vi "SelfCal.vi"(8 "error in (no error)":errorcluster, 10 "gRPCid":T4, 11 "ctet_smu":T1) -> (0 "error out":errorcluster, 3 "ctet_smu out":T1)   [LabVIEW 2019, in "ctet_smu User Library.lvlib"]
uses:
  ctet_smu User Library.lvlib
  Servers/ctet_smu/gRPC lvSupport/Server API/typeDefs/grpcId.ctl
  Types/ctet_smu.ctl
  Servers/ctet_smu/ctet_smu Class/RPC Messages/measurementservice_SMUConfigResponse/measurementservice_SMUConfigResponse_Data.ctl
  Servers/ctet_smu/ctet_smu Class/RPC Messages/measurementservice_ErrorOut/measurementservice_ErrorOut_Data.ctl
  Servers/ctet_smu/ctet_smu Class/RPC Messages/measurementservice_SMUSelfCalResponse/measurementservice_SMUSelfCalResponse_Data.ctl
  Servers/ctet_smu/ctet_smu Class/ctet_smu.lvclass
  Servers/ctet_smu/gRPC lvSupport/gprc-lvsupport.lvlib
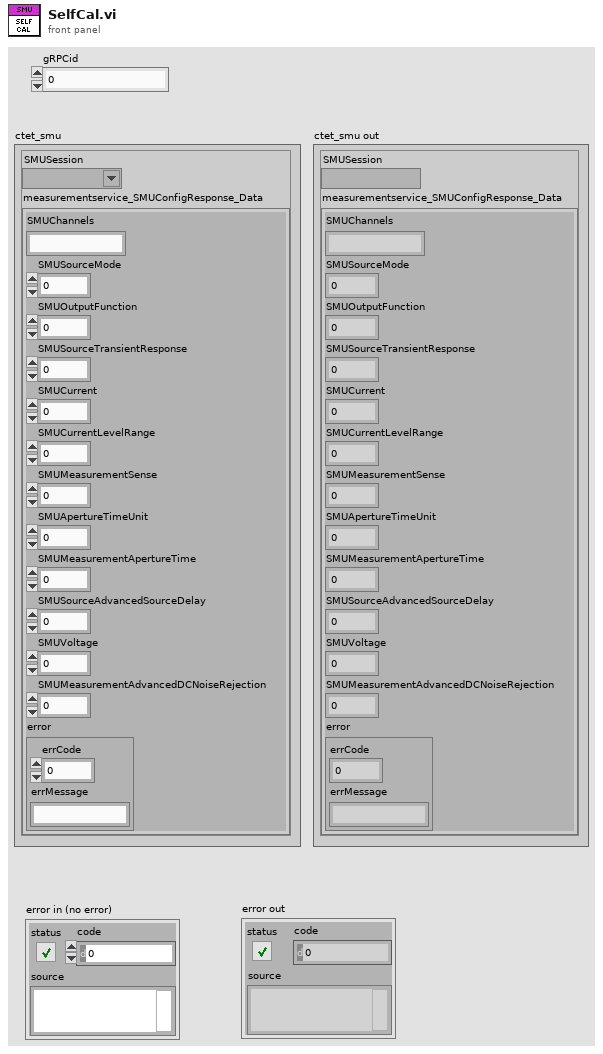
[diagram p1: front panel]
types:
  T1 = typedef "ctet_smu User Library.lvlib/ctet_smu.ctl" = cluster{"SMUSession":refnum<k15>, "measurementservice_SMUConfigResponse_Data":T2}
  T2 = typedef "ctet_smu.lvlib/ctet_smu.lvclass/measurementservice_SMUConfigResponse_Data.ctl" = cluster{"SMUChannels":string, "SMUSourceMode":i64, "SMUOutputFunction":i64, "SMUSourceTransientResponse":i64, "SMUCurrent":dbl, "SMUCurrentLevelRange":dbl, "SMUMeasurementSense":i64, "SMUApertureTimeUnit":i64, "SMUMeasurementApertureTime":dbl, "SMUSourceAdvancedSourceDelay":dbl, "SMUVoltage":dbl, "SMUMeasurementAdvancedDCNoiseRejection":i64, "error":T3}
  T3 = typedef "ctet_smu.lvlib/ctet_smu.lvclass/measurementservice_ErrorOut_Data.ctl" = cluster{"errCode":i64, "errMessage":string}
  T4 = typedef "ctet_smu.lvlib/gprc-lvsupport.lvlib/grpcId.ctl" = u64
  T5 = typedef "ctet_smu.lvlib/ctet_smu.lvclass/measurementservice_SMUSelfCalResponse_Data.ctl" = cluster{"error":T3}
  T6 = typedef "ctet_smu.lvlib/ctet_smu.lvclass/measurementservice_SMUSelfCalRequest_Data.ctl" = cluster{"SMUName":string, "SMUChannels":string}
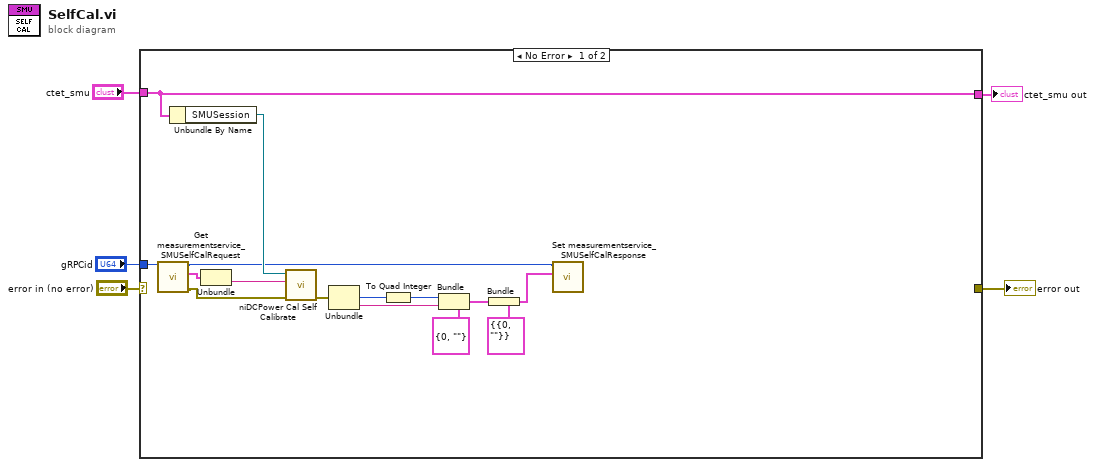
[diagram p0: block diagram]
diagram:
  n1 = case shown="No Error" "error in (no error)" {
    selector: "error in (no error)" -> [_ w22]
    tunnel: [_ w22] -> w5
    tunnel: "gRPCid" -> [w14 _]
    tunnel: "ctet_smu" -> [w15 w21]
    tunnel: [w15 w21] -> w1
    frame No Error {
      n2 = call "Get measurementservice_SMUSelfCalRequest.vi"("gRPCid"=w14) -> ("error out"=w13:errorcluster, "Message Data"=w12:T6, "gRPCid out"=w10:T4)  [unwired: 8 in]
      n3 = Unbundle By Name(w15) -> ("SMUSession"=w16:refnum<k15>)
      n4 = Unbundle(w12) -> ("SMUChannels"=w11:string)  [unwired: 1 out]
      n5 = call <instrlib>:"niDCPower Cal Self Calibrate.vi"("error in (no error)"=w13, "channel name"=w11, "instrument handle"=w16) -> ("error out"=w20:errorcluster)  [unwired: 7 in, 1 out]
      n6 = Unbundle(w20) -> ("code"=w18:i32, "source"=w19:string)  [unwired: 1 out]
      n7 = To Quad Integer(1:w18) -> (0:w17:i64)
      n8 = Bundle(cluster=T3 {"errCode"=0, "errMessage"=""} ("error"), "errCode"=w17, "errMessage"=w19) -> (w7:T3)
      n9 = Bundle(cluster=T5 {"error"={"errCode"=0, "errMessage"=""}} ("measurementservice_SMUSelfCalResponse_Data"), "error"=w7) -> (w6:T5)
      n10 = call "Set measurementservice_SMUSelfCalResponse.vi"("Message Data"=w6, "gRPCid"=w10) -> ()  [unwired: 9 in, 1 out]
    }
    frame Error {
    }
  }
  "error out" <- w5
  "ctet_smu out" <- w1
